vi "DB FGV.vi"(8 "error in":errorcluster, 9 "Action":enum16{"Get", "Set"}(ring), 10 "connection reference":T1, 11 "Database.lvclass":refnum<class "Database.lvclass">) -> (0 "error out":errorcluster, 2 "connection reference Out":T1, 3 "Database Out.lvclass":refnum<class "Database.lvclass">)   [LabVIEW 2023, in "HardwareAbstractionLayer_LVOOP.lvlib" / "Database.lvclass"]
uses:
  Database.lvclass
  <vilib>/addons/database/Connection.llb/Conn ObjectReference.ctl
  <vilib>/addons/database/NI_Database_API.lvlib
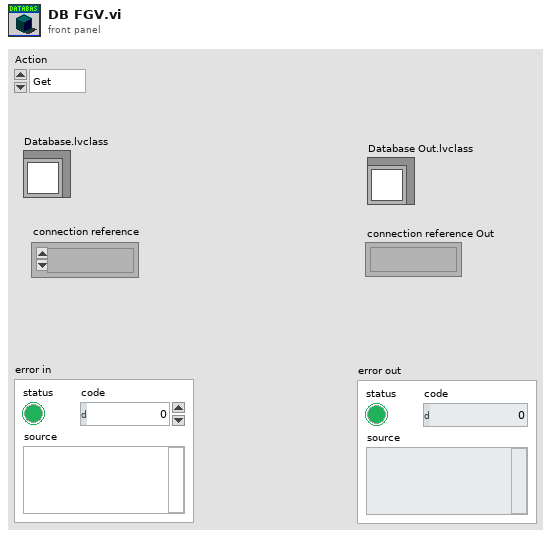
[diagram p1: front panel]
types:
  T1 = typedef "NI_Database_API.lvlib/Conn ObjectReference.ctl" = refnum<k1>
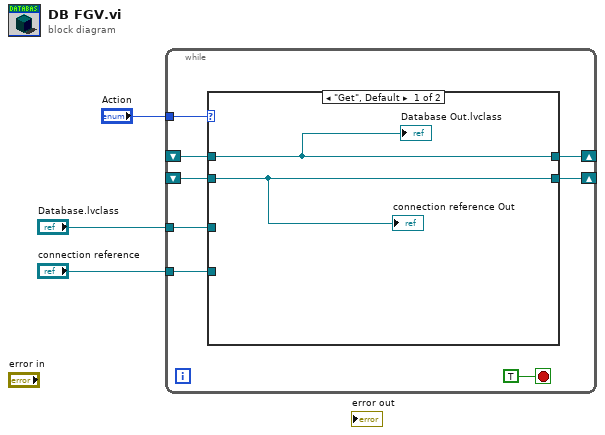
[diagram p0: block diagram]
diagram:
  n1 = while {
    shift-right: [w7] -> _
    shift-left: _ -> [w10]
    tunnel: "Action" -> [w9]
    tunnel: "Database.lvclass" -> [w8]
    tunnel: "connection reference" -> [w6]
    shift-right: [w5] -> _
    shift-left: _ -> [w4]
    stop <- TRUE stop-if-true
    n2 = case shown="\"Get\", Default" w9 {
      tunnel: w10 -> [w13 _]
      tunnel: w8 -> [_ w15]
      tunnel: [w13 w15] -> w7
      tunnel: w6 -> [_ w14]
      tunnel: [w12 w14] -> w5
      tunnel: w4 -> [w12 _]
      frame "Get", Default {
        "Database Out.lvclass" <- w13
        "connection reference Out" <- w12
      }
      frame "Set" {
      }
    }
  }
